vi "Global_CMD_CMD_Data In.vi"() -> ()   [LabVIEW 2020, in "2023-Auto_CMD.lvlib"]
uses:
  2023-Auto_CMD.lvlib
  Cluster_CMD_CMD_Data.ctl
  Shared Code/TypeDefs/ENUM_AutoSelect.ctl
panel:
  in  "CMD_CMD_2022-Auto_Data":T1={"Auto Select"=enum."Drop High dock and engage"}
  # "The Names of the Data items in the Global Variable MUST describe who the Single Writer is\nFor Command Globals the Commander(CMD) represents Teleop or Autonomous or other command loop.\nThe naming convention for a Command for a Command Global is:   \n\nCMD_CMD_LibName_Data Name\n\nExample:\nCMD_CMD_BallShooter_Data\nCMD_CMD_ProgramedMotion1_Data"
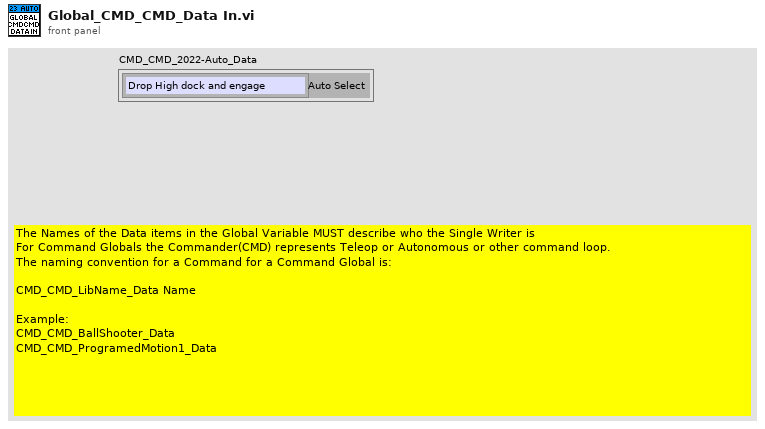
[diagram p1: front panel]
types:
  T1 = typedef "2023-Auto_CMD.lvlib/Cluster_CMD_CMD_Data.ctl" = cluster{"Auto Select":T2}
  T2 = typedef "ENUM_AutoSelect.ctl" = enum16{"Unknown", "Drop High Drive Straight", "Drop mid dock and engage", "Drop High dock and engage", "Auto 4", "Manual"}
diagram:
